vi "conTrig.vi"(3 "error in":errorcluster, 4 "Voltage Scale":dbl(ring)=2.0 items=["8 V"=8.0, "4 V"=4.0, "2 V"=2.0, "800 mV"=0.8, "400 mV"=0.4, "200 mV"=0.2, "80 mV"=0.08], 5 "Trigger":T1 {"Slope" items=["Positive", "Negative"]; "Level" format="%.2f"; "Coupling" items=["DC 1 MOhm", "AC 1 MOhm", "DC 50 Ohm", "AC 50 Ohm"]; "Source" items=["Chan 1", "External"]}, 6 "InstrumentID":u32) -> (0 "error out":errorcluster, 2 "dup id":u32 format="%.0x")   [LabVIEW 2022 SP3]
uses:
  <instrlib>/Acqiris Dx/Acqiris Dx.lvlib
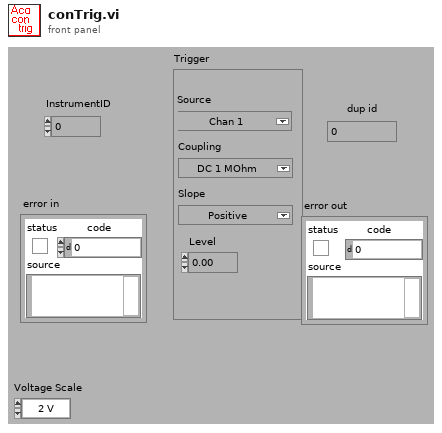
[diagram p1: front panel]
types:
  T1 = cluster{"Source":u16, "Coupling":u16, "Slope":u16, "Level":dbl}
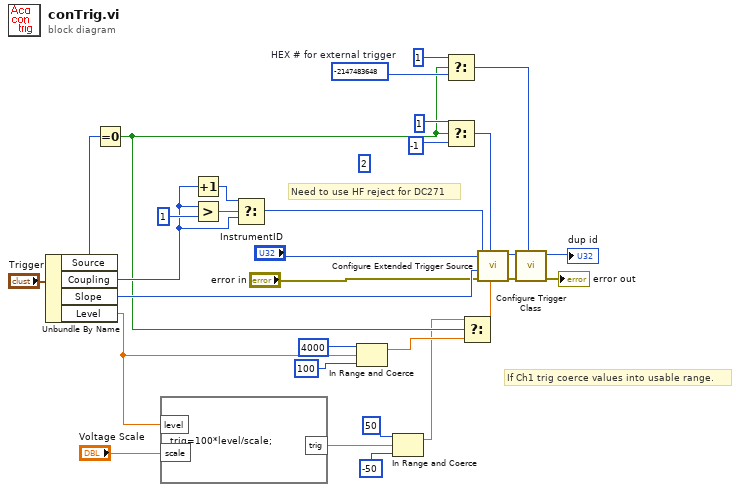
[diagram p0: block diagram]
diagram:
  (unwired) 2
  w30 = -2147483648  # HEX # for external trigger
  # "If Ch1 trig coerce values into usable range."
  # "Need to use HF reject for DC271"
  n1 = Unbundle By Name("Trigger") -> ("Source"=w23:u16, "Coupling"=w25:u16, "Slope"=w29:u16, "Level"=w4:dbl)
  n2 = Equal To 0?(x=w23) -> (x = 0?=w14:bool)
  n3 = formula code="trig=100*level/scale;"("level"=w4, "scale"="Voltage Scale") -> ("trig"=w3:dbl)
  n4 = Increment(x=w25) -> (x+1=w26:u16)
  n5 = Greater?(x=w25, y=1) -> (0:w27:bool)
  n6 = Select(t=w26, s=w27, f=w25) -> (s? t:f=w7:u16)
  n7 = In Range and Coerce(upper limit=4000, x=w4, lower limit=100) -> (coerced(x)=w10:dbl)  [unwired: 1 out]
  n8 = In Range and Coerce(upper limit=50, x=w3, lower limit=-50) -> (coerced(x)=w2:dbl)  [unwired: 1 out]
  n9 = Select(t=1, s=w14, f=w30) -> (s? t:f=w31:i32)
  n10 = Select(t=1, s=w14, f=-1) -> (s? t:f=w22:i32)
  n11 = Select(t=w2, s=w14, f=w10) -> (s? t:f=w13:dbl)
  n12 = call <instrlib>:"Configure Extended Trigger Source.vi"("Trigger Level 1 (0)"=w13, "Channel (1)"=w22, "error in (no error)"="error in", "Trigger Slope (0: positive)"=w29, "Trigger Coupling (0: DC)"=w7, "Instrument ID"="InstrumentID") -> ("error out"=w20:errorcluster, "dup Instrument ID"=w19:u32)  [unwired: 1 in, 3 out]
  n13 = call <instrlib>:"Configure Trigger Class.vi"("Source Pattern (1: Chan 1)"=w31, "error in (no error)"=w20, "Instrument ID"=w19) -> ("error out"=→"error out":errorcluster, "dup Instrument ID"=→"dup id":u32)  [unwired: 1 in, 6 out]
